vi "CCE RRMA P01 SubVI02.vi"(11 "Array":u32[][](array[numeric])) -> (2 "cy":u32, 3 "cx":u32)   [LabVIEW 2020]
doc: "Ceballos Conde Emanuel Rodríguez Ramírez Miguel Ángel 4MV6 Sistemas de visión artificial 2022/1\nEste vi permite obtener al centroide de una imagen representada por un arreglo de 2 dimensiones , el centroide obtenido es dado respecto al origen de la imagen (esquina superior izquierda)"
panel:
  out "fx":dbl[](array[numeric])
  out "fy":dbl[](array[numeric])
  out "x":dbl[](array[numeric])
  out "size(s)":i32[](array[numeric])
  out "y":dbl[](array[numeric])
  # "Ceballos Conde Emanuel\nRodríguez Ramírez Miguel Ángel\n4MV6\nSistemas de visión artificial\n2022/1"
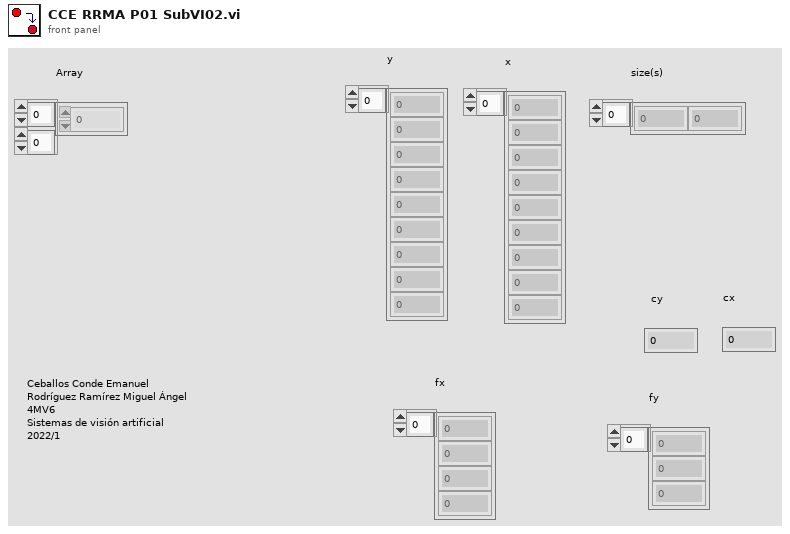
[diagram p1: front panel]
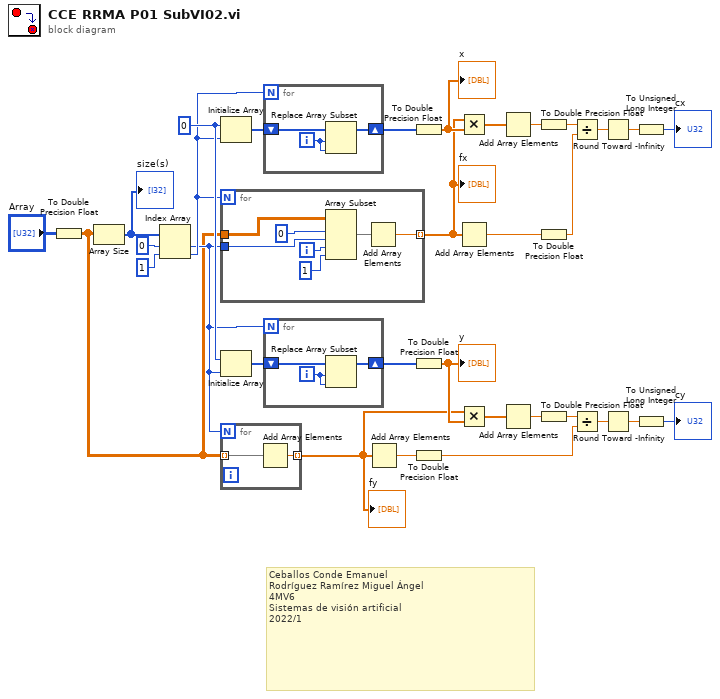
[diagram p0: block diagram]
diagram:
  w30 = 0 ("index")
  # "Ceballos Conde Emanuel\nRodríguez Ramírez Miguel Ángel\n4MV6\nSistemas de visión artificial\n2022/1"
  n1 = To Double Precision Float(number="Array") -> (double precision float=w2:dbl[][])
  n2 = Array Size(array=w2) -> (size(s)=w24:i32[])
  "size(s)" <- w24
  n3 = Index Array(array=w24, index #1=0 ("index"), index #2=1 ("index")) -> (element #1=w26:i32, element #2=w27:i32)
  n4 = Initialize Array(w30, w27) -> (w29:i32[])
  n5 = for {
    N: w27 -> [_]
    tunnel: w2 -> [w39]
    tunnel: w26 -> [w37]
    tunnel: [w33] -> w20 mode=indexing
    i -> [w36]
    n6 = Array Subset(array=w39, index (row)=0 ("index"), length (row)=w37, index (col)=w36, length (col)=1 ("length")) -> (w34:dbl[][])
    n7 = Add Array Elements(numeric array=w34) -> (sum=w33:dbl)
  }
  "fx" <- w20
  n8 = Initialize Array(w30, w26) -> (w28:i32[])
  n9 = for {
    N: w26 -> [_]
    tunnel: w2 -> [w41] mode=indexing
    tunnel: [w40] -> w1 mode=indexing
    n10 = Add Array Elements(numeric array=w41) -> (sum=w40:dbl)
  }
  "fy" <- w1
  n11 = for {
    N: w27 -> [_]
    shift-right: [w42] -> w25
    shift-left: w29 -> [w44]
    i -> [w43]
    n12 = Replace Array Subset(array=w44, new element=w43, index=w43) -> (w42:i32[])
  }
  n13 = for {
    N: w26 -> [_]
    shift-right: [w46] -> w9
    shift-left: w28 -> [w45]
    i -> [w47]
    n14 = Replace Array Subset(array=w45, new element=w47, index=w47) -> (w46:i32[])
  }
  n15 = Add Array Elements(numeric array=w1) -> (sum=w13:dbl)
  n16 = To Double Precision Float(number=w25) -> (double precision float=w23:dbl[])
  "x" <- w23
  n17 = To Double Precision Float(number=w9) -> (double precision float=w8:dbl[])
  "y" <- w8
  n18 = To Double Precision Float(number=w13) -> (double precision float=w11:dbl)
  n19 = Multiply(x=w20, y=w23) -> (x*y=w22:dbl[])
  n20 = Add Array Elements(numeric array=w20) -> (sum=w19:dbl)
  n21 = Multiply(x=w1, y=w8) -> (x*y=w15:dbl[])
  n22 = Add Array Elements(numeric array=w22) -> (sum=w21:dbl)
  n23 = Add Array Elements(numeric array=w15) -> (sum=w14:dbl)
  n24 = To Double Precision Float(number=w21) -> (double precision float=w16:dbl)
  n25 = To Double Precision Float(number=w19) -> (double precision float=w17:dbl)
  n26 = To Double Precision Float(number=w14) -> (double precision float=w10:dbl)
  n27 = Divide(x=w16, y=w17) -> (x/y=w18:dbl)
  n28 = Divide(x=w10, y=w11) -> (x/y=w12:dbl)
  n29 = Round Toward -Infinity(1:w18) -> (0:w6:dbl)
  n30 = Round Toward -Infinity(1:w12) -> (0:w7:dbl)
  n31 = To Unsigned Long Integer(number=w6) -> (unsigned 32bit integer=→"cx":u32)
  n32 = To Unsigned Long Integer(number=w7) -> (unsigned 32bit integer=→"cy":u32)
